vi "ArduinoIO.vi"() -> ()   [LabVIEW 2014]
uses:
  <vilib>/Instr/_visa.llb/VISA Configure Serial Port (Instr).vi
panel:
  out "Vmot":dbl
  out "Yaw angle":dbl
  out "RPM":dbl
  in  "Counts / rev":u32
  in  "Flush?":bool
  out "read buffer":string
  in  "stop":bool
  in  "VISA resource name":refnum<visa-resource-name>
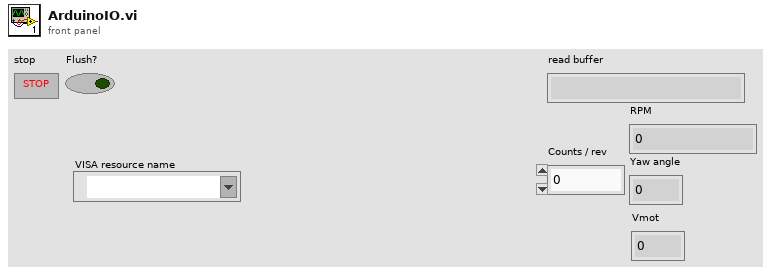
[diagram p1: front panel]
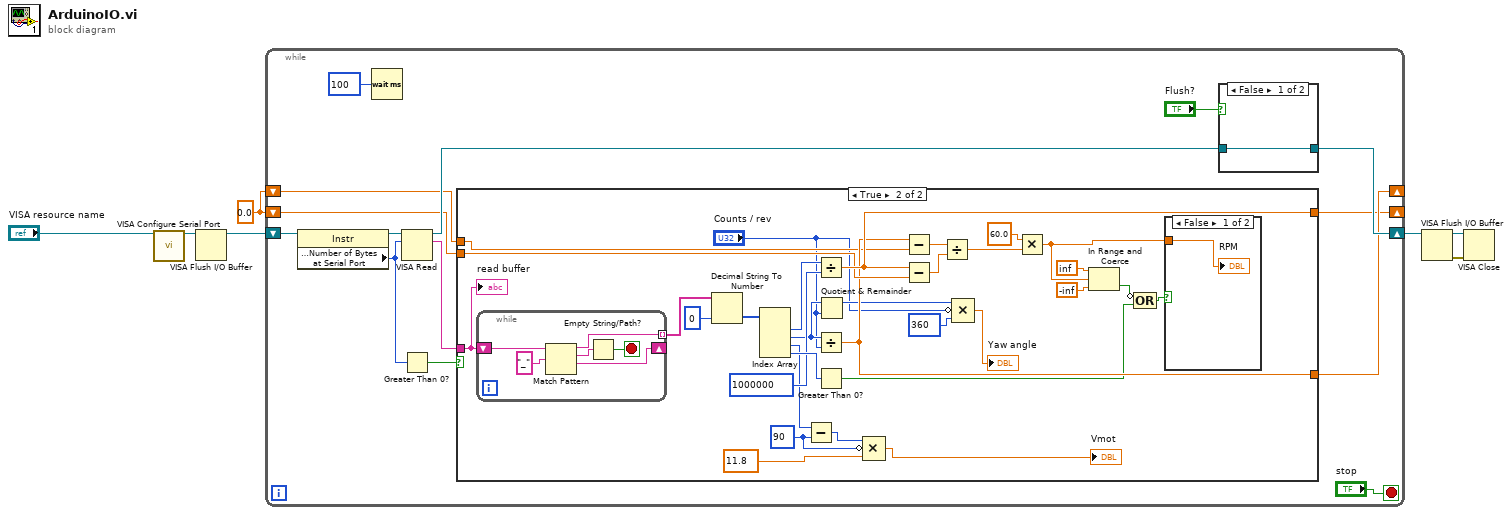
[diagram p0: block diagram]
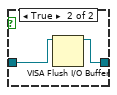
[diagram p4: hidden frame]
diagram:
  w1 = 0.0
  n1 = call-poly "VISA Configure Serial Port"("VISA resource name"="VISA resource name") -> ("VISA resource name out"=w3:refnum<visa-resource-name>)  [unwired: 13 in, 1 out]
  n2 = VISA Flush I/O Buffer(VISA resource name=w3) -> (VISA resource name out=w2:refnum<visa-resource-name>)  [unwired: 2 in, 1 out]
  n3 = while {
    shift-right: [w16] -> w5
    shift-left: w2 -> [w18]
    shift-right: [w9] -> _
    shift-left: w1 -> [w11]
    shift-right: [w8] -> _
    shift-left: w1 -> [w10]
    stop <- "stop" stop-if-true
    n4 = property class="Instr"(reference=w18) -> (reference out=w20:refnum<visa-resource-name>, "Serial Settings:Number of Bytes at Serial Port"=w14:u32)  [unwired: 1 in, 1 out]
    n5 = Wait (ms)(milliseconds to wait=u32 100) -> ()  [unwired: 1 out]
    n6 = VISA Read(VISA resource name=w20, byte count=w14) -> (VISA resource name out=w17:refnum<visa-resource-name>, read buffer=w12:string)  [unwired: 1 in, 2 out]
    n7 = Greater Than 0?(x=w14) -> (x > 0?=w13:bool)
    n8 = case shown="True" w13 {
      tunnel: w12 -> [_ w54]
      tunnel: w11 -> [w23 w44]
      tunnel: w10 -> [w22 w46]
      tunnel: [w23 w45] -> w9
      tunnel: [w22 w47] -> w8
      frame False {
      }
      frame True {
        w26 = u32 90 ("y")
        n9 = while {
          shift-right: [w59] -> _
          shift-left: w54 -> [w61]
          tunnel: [w56] -> w53 mode=indexing
          stop <- w57 stop-if-true
          n10 = Match Pattern(string=w61, regular expression="_") -> (before substring=w56:string, match substring=w58:string, after substring=w59:string)  [unwired: 1 in, 1 out]
          n11 = Empty String/Path?(string/path=w58) -> (empty?=w57:bool)
        }
        n12 = Decimal String To Number(string=w53, default (0L)=u32 0) -> (number=w51:u32[])  [unwired: 1 in, 1 out]
        n13 = Index Array(array=w51) -> (element #1=w49:u32, element #2=w35:u32, element #3=w28:u32, element #4=w50:u32)  [unwired: 4 in]
        n14 = Subtract(x=w28, y=w26) -> (x-y=w27:u32)
        n15 = Divide(x=w49, y=u32 1000000) -> (x/y=w47:dbl)
        n16 = Divide(x=w35, y="Counts / rev") -> (x/y=w45:dbl)
        n17 = Greater Than 0?(x=w50) -> (x > 0?=w29:bool)
        n18 = Quotient & Remainder(x=w35, y="Counts / rev") -> (x-y*floor(x/y)=w34:u32)  [unwired: 1 out]
        n19 = Compound Arithmetic op=MULTIPLY(w27, invert w26, 11.8 ("value")) -> (→"Vmot":dbl)
        n20 = Subtract(x=w45, y=w44) -> (x-y=w42:dbl)
        n21 = Subtract(x=w47, y=w46) -> (x-y=w43:dbl)
        n22 = Divide(x=w42, y=w43) -> (x/y=w41:dbl)
        n23 = Compound Arithmetic op=MULTIPLY(w34, invert "Counts / rev", u32 360 ("value")) -> (→"Yaw angle":dbl)
        n24 = Multiply(x=60.0, y=w41) -> (x*y=w36:dbl)
        n25 = In Range and Coerce(upper limit=inf, x=w36, lower limit=-inf) -> (In Range?=w30:bool)  [unwired: 1 out]
        n26 = Compound Arithmetic op=OR(invert w30, w29) -> (w39:bool)
        n27 = case shown="False" w39 {
          tunnel: w36 -> [w55 _]
          frame False {
            "RPM" <- w55
          }
          frame True {
          }
        }
        "read buffer" <- w54
      }
    }
    n28 = case shown="False" "Flush?" {
      tunnel: w17 -> [w62 w64]
      tunnel: [w62 w63] -> w16
      frame False {
      }
      frame True {
        n29 = VISA Flush I/O Buffer(VISA resource name=w64) -> (VISA resource name out=w63:refnum<visa-resource-name>)  [unwired: 2 in, 1 out]
      }
    }
  }
  n30 = VISA Flush I/O Buffer(VISA resource name=w5) -> (VISA resource name out=w6:refnum<visa-resource-name>, error out=w7:errorcluster)  [unwired: 2 in]
  n31 = VISA Close(VISA resource name=w6, error in (no error)=w7) -> ()  [unwired: 1 out]
